vi "Helper_Distance_Two_Points.vi"(1 "y 2":dbl, 2 "x 2":dbl, 3 "y":dbl, 4 "x":dbl) -> (0 "Numeric":dbl)   [LabVIEW 2011]
panel:
  # "Point 1"
  # "Point 2"
  # "Difference between Points"
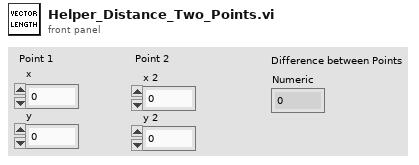
[diagram p1: front panel]
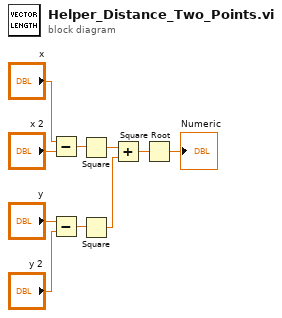
[diagram p0: block diagram]
diagram:
  n1 = Subtract(x="x", y="x 2") -> (x-y=w6:dbl)
  n2 = Subtract(x="y", y="y 2") -> (x-y=w5:dbl)
  n3 = Square(x=w6) -> (x^2=w7:dbl)
  n4 = Square(x=w5) -> (x^2=w8:dbl)
  n5 = Add(x=w7, y=w8) -> (x+y=w9:dbl)
  n6 = Square Root(x=w9) -> (sqrt(x)=→"Numeric":dbl)
